vi "Pre Launch Init.vi"(11 "RootModelPublishesDoubleFloat In":refnum<class "RootModelPublishesDoubleFloat.lvclass">) -> (0 "error out":errorcluster, 3 "RootModelPublishesDoubleFloat Out":refnum<class "RootModelPublishesDoubleFloat.lvclass">)   [LabVIEW 2017, in "RootModelPublishesDoubleFloat.lvlib" / "RootModelPublishesDoubleFloat.lvclass"]
doc: "(<B>Filename</B>: Actor Framework.lvlib:Actor.lvclass:Pre Launch Init.vi)\n\nDefines behavior that occurs after the Launch Nested Actor method is invoked but before the actor's Actor Core method begins running.\n\nBy default, this method does nothing. A descendant class may override it to define behavior."
uses:
  RootModelPublishesDoubleFloat.lvclass
  C:/Program Files (x86)/National Instruments/LabVIEW 2017/vi.lib/ActorFramework/Actor/Actor.lvclass
  <vilib>/ActorFramework/Actor/Actor.lvclass/Actor.ctl
  <vilib>/ActorFramework/Message Enqueuer/Message Enqueuer.lvclass/Message Enqueuer.ctl
  <vilib>/ActorFramework/Message Enqueuer/Init from Existing Queue.vi
  <vilib>/ActorFramework/Message Enqueuer/Enqueue.vi
  RootModelPublishesDoubleFloat Messages/Publish Test Value Msg/Publish Test Value Msg.lvclass
  C:/Program Files (x86)/National Instruments/LabVIEW 2017/vi.lib/ActorFramework/Message/Message.lvclass
  <vilib>/ActorFramework/Message Priority Queue/Priority Enqueue.vi
  Source/RootModel/RootModel/RootModel.lvclass
  <vilib>/ActorFramework/Message Enqueuer/Message Enqueuer.lvclass
  <vilib>/ActorFramework/Actor/Actor.lvclass
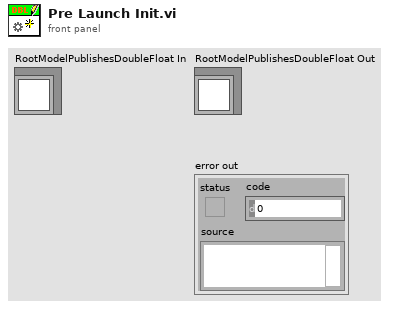
[diagram p1: front panel]
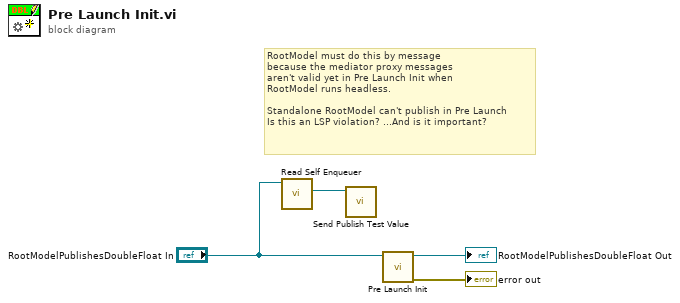
[diagram p0: block diagram]
diagram:
  # "RootModel must do this by message\nbecause the mediator proxy messages\naren't valid yet in Pre Launch Init when\nRootModel runs headless.\n\nStandalone RootModel can't publish in Pre Launch\nIs this an LSP violation? ...And is it important?"
  n1 = call <vilib>:"Read Self Enqueuer.vi"("Actor"="RootModelPublishesDoubleFloat In") -> ("Self Enqueuer"=w1:refnum<class "Message Enqueuer.lvclass">)  [unwired: 10 in]
  n2 = call "Send Publish Test Value.vi"("Message Enqueuer"=w1) -> ()  [unwired: 9 in, 2 out]
  n3 = call-parent "Pre Launch Init.vi"("RootModel in"="RootModelPublishesDoubleFloat In") -> ("error out"=→"error out":errorcluster, "RootModel out"=→"RootModelPublishesDoubleFloat Out":refnum<class "RootModelPublishesDoubleFloat.lvclass">)  [unwired: 9 in]
